vi "Scale Image.vi"(8 "error in (no error)":errorcluster, 9 "Path":path, 10 "New Dimensions":cluster{"Width":i32, "Height":i32}, 11 "Image":refnum<k24>) -> (0 "error out":errorcluster, 3 "Scaled Image":T1)   [LabVIEW 2020, in "MacroAssert.lvlib" / "Win Util.lvlib"]
doc: "This VI will use window refnum in to get the name of a window. The name of a window is simply the text appearing in the title bar of the window. If the title bar of the window is not shown, the name of the window will be a NULL string."
uses:
  Win Util.lvlib
  <vilib>/picture/picture.llb/imagedata.ctl
  System.Drawing
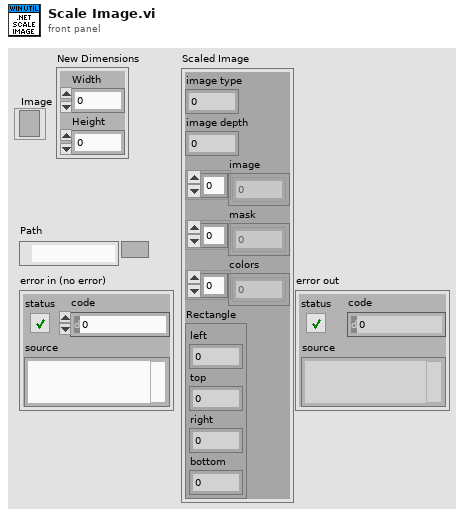
[diagram p1: front panel]
types:
  T1 = typedef "imagedata.ctl" = cluster{"image type":i32, "image depth":i32, "image":u8[], "mask":u8[], "colors":u32[], "Rectangle":cluster{"left":i16, "top":i16, "right":i16, "bottom":i16}}
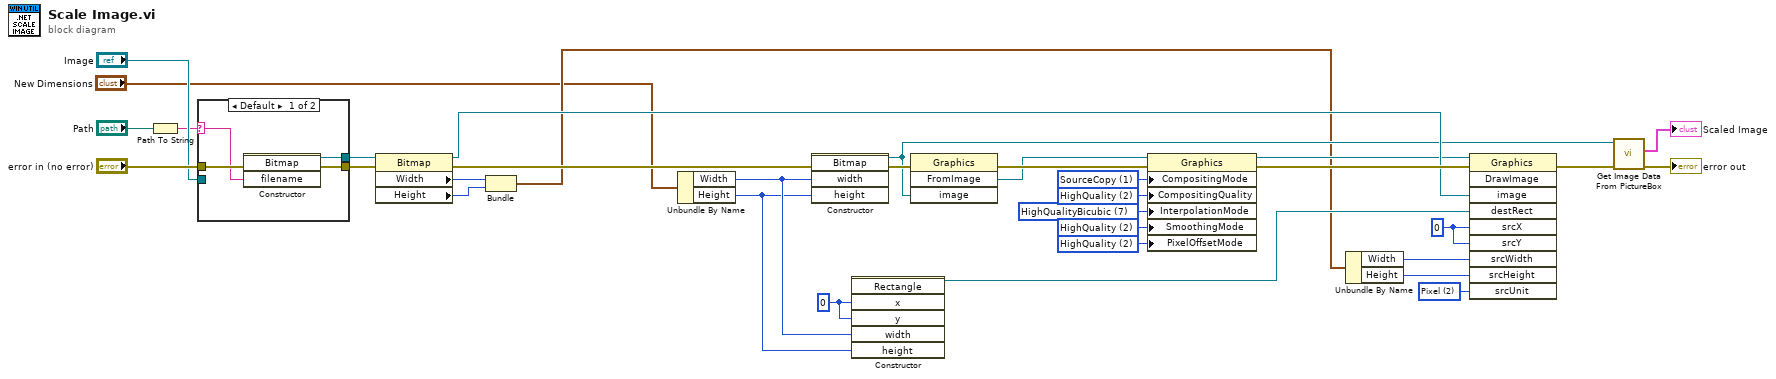
[diagram p0: block diagram]
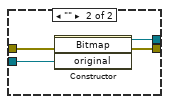
[diagram p2: hidden frame]
diagram:
  w5 = 2 items=["World", "Display", "Pixel", "Point", "Inch", "Document", "Millimeter"] ("srcUnit")
  w9 = 0 ("srcX")
  w10 = 2 items=["Default"=0, "HighSpeed"=1, "HighQuality"=2, "None"=3, "Half"=4, "Invalid"=-1] ("PixelOffsetMode")
  w11 = 2 items=["Default"=0, "HighSpeed"=1, "HighQuality"=2, "None"=3, "AntiAlias"=4, "Invalid"=-1] ("SmoothingMode")
  w12 = 7 items=["Default"=0, "Low"=1, "High"=2, "Bilinear"=3, "Bicubic"=4, "NearestNeighbor"=5, "HighQualityBilinear"=6, "HighQualityBicubic"=7, "Invalid"=-1] ("InterpolationMode")
  w13 = 2 items=["Default"=0, "HighSpeed"=1, "HighQuality"=2, "GammaCorrected"=3, "AssumeLinear"=4, "Invalid"=-1] ("CompositingQuality")
  w14 = 1 items=["SourceOver", "SourceCopy"] ("CompositingMode")
  w15 = 0 ("x")
  n1 = Path To String(path="Path") -> (string=w19:string)
  n2 = case shown="Default" w19 {
    selector: w19 -> [w35 _]
    tunnel: [w36 w40] -> w26
    tunnel: [w38 w42] -> w30
    tunnel: "error in (no error)" -> [w37 w41]
    tunnel: "Image" -> [_ w39]
    frame Default {
      n3 = constructor class="Bitmap"(error in=w37, "filename"=w35) -> (reference out=w36:refnum<k24>, error out=w38:errorcluster)  [unwired: 2 in, 2 out]
    }
    frame "" {
      n4 = constructor class="Bitmap"(error in=w41, "original"=w39) -> (reference out=w40:refnum<k24>, error out=w42:errorcluster)  [unwired: 2 in, 2 out]
    }
  }
  n5 = property class="Bitmap"(reference=w26, error in=w30) -> (reference out=w24:refnum<k24>, error out=w27:errorcluster, "Width"=w18:i32, "Height"=w17:i32)
  n6 = Bundle("Width"=w18, "Height"=w17) -> (w8:cluster{"Width":i32, "Height":i32})  [unwired: 1 in]
  n7 = Unbundle By Name("New Dimensions") -> ("Width"=w16:i32, "Height"=w3:i32)
  n8 = constructor class="Bitmap"(error in=w27, "width"=w16, "height"=w3) -> (reference out=w21:refnum<k24>, error out=w34:errorcluster)  [unwired: 2 in, 3 out]
  n9 = constructor class="Rectangle"("x"=w15, "y"=w15, "width"=w16, "height"=w3) -> (reference out=w23:refnum<k24>)  [unwired: 3 in, 6 out]
  n10 = invoke class="Graphics" method="FromImage"(error in=w34, "image"=w21) -> (error out=w33:errorcluster, "FromImage"=w25:refnum<k24>)  [unwired: 2 in, 2 out]
  n11 = property class="Graphics"(reference=w25, error in=w33, "CompositingMode"=w14, "CompositingQuality"=w13, "InterpolationMode"=w12, "SmoothingMode"=w11, "PixelOffsetMode"=w10) -> (reference out=w22:refnum<k24>, error out=w32:errorcluster)
  n12 = Unbundle By Name(w8) -> ("Width"=w7:i32, "Height"=w6:i32)
  n13 = invoke class="Graphics" method="DrawImage"(reference=w22, error in=w32, "image"=w24, "destRect"=w23, "srcX"=w9, "srcY"=w9, "srcWidth"=w7, "srcHeight"=w6, "srcUnit"=w5) -> (error out=w31:errorcluster)  [unwired: 1 in, 9 out]
  n14 = call "Get Image Data From PictureBox.vi"("error in (no error)"=w31, "Image"=w21) -> ("error out"=→"error out":errorcluster, "Image Data"=→"Scaled Image":T1)  [unwired: 7 in, 1 out]
